vi "Stay when Set.vi"() -> ()   [LabVIEW 2009]
panel:
  in  "stop":bool
  in  "Reset":bool
  out "Trigger":bool
  in  "Signal":bool
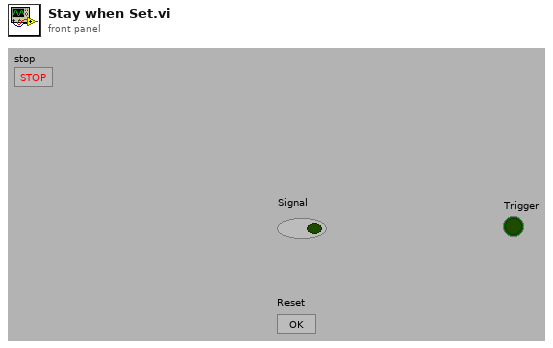
[diagram p1: front panel]
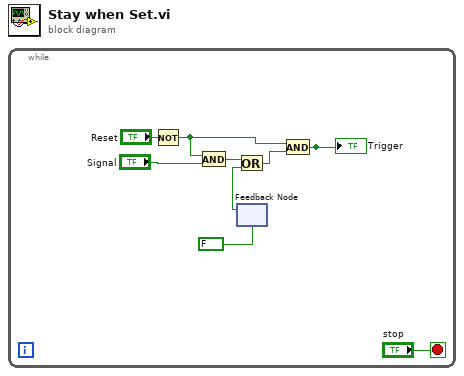
[diagram p0: block diagram]
diagram:
  n1 = while {
    stop <- "stop" stop-if-true
    n2 = Not(x="Reset") -> (.not. x?=w2:bool)
    n3 = And(x=w2, y="Signal") -> (x .and. y?=w3:bool)
    n4 = feedback #1(FALSE) -> (w9:bool)
    n5 = Or(x=w3, y=w9) -> (x .or. y?=w5:bool)
    n6 = And(x=w2, y=w5) -> (x .and. y?=w4:bool)
    "Trigger" <- w4
  }
